vi "Clear.vi"(8 "error in (no error)":errorcluster, 11 "Error Handler In":refnum<class "Error Handler.lvclass">) -> (0 "error out":errorcluster, 3 "Error Handler Out":refnum<class "Error Handler.lvclass">)   [LabVIEW 2020, in "Error Handler.lvclass"]
uses:
  Error Handler.lvclass
  Error Handler.lvclass/Error Handler.ctl
  Process/Process.lvclass
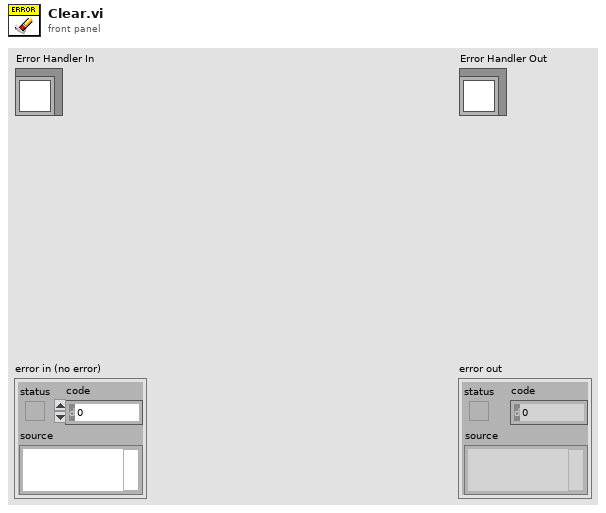
[diagram p1: front panel]
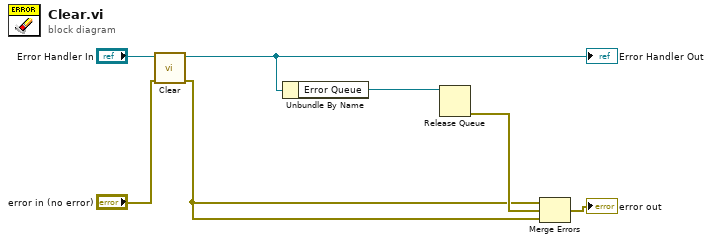
[diagram p0: block diagram]
diagram:
  n1 = call-parent "Clear.vi"("error in (no error)"="error in (no error)", "Process In"="Error Handler In") -> ("error out"=w1:errorcluster, "Process Out"=w2:refnum<class "Error Handler.lvclass">)  [unwired: 8 in]
  "Error Handler Out" <- w2
  n2 = Unbundle By Name(w2) -> ("Error Queue"=w5:refnum<queue>)
  n3 = Release Queue(queue=w5) -> (error out=w4:errorcluster)  [unwired: 2 in, 2 out]
  n4 = Merge Errors(w1, w4, w1) -> (→"error out":errorcluster)
